vi "ReadTriggered.vi"(8 "error in (no error)":errorcluster, 10 "Keep last record only":bool, 11 "Scope5785_six_channel":refnum<class "Scope5782_six_channel.lvclass">) -> (0 "error out":errorcluster, 1 "#elements":i32, 2 "Data":dbl[][](array[numeric]), 3 "Scope5785_six_channel Out":refnum<class "Scope5782_six_channel.lvclass">)   [LabVIEW 2018, in "Scope5782_six_channel.lvclass"]
uses:
  Scope5782_six_channel.lvclass
  FpgaRef/FpgaRef5761/FpgaRef5761.lvclass
  FpgaRef/FpgaRef5782/FpgaRef5782.lvclass
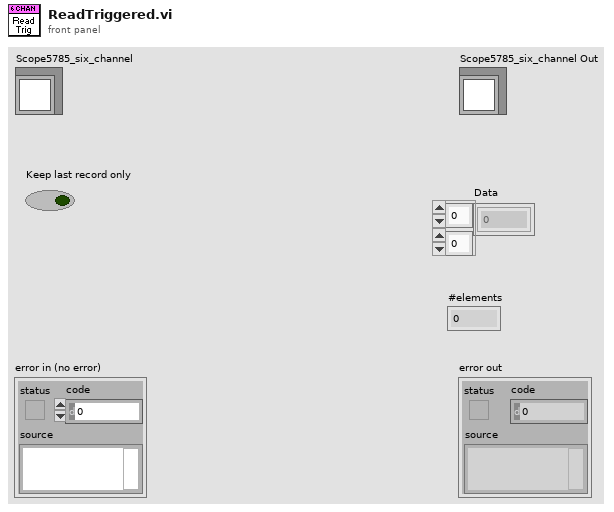
[diagram p1: front panel]
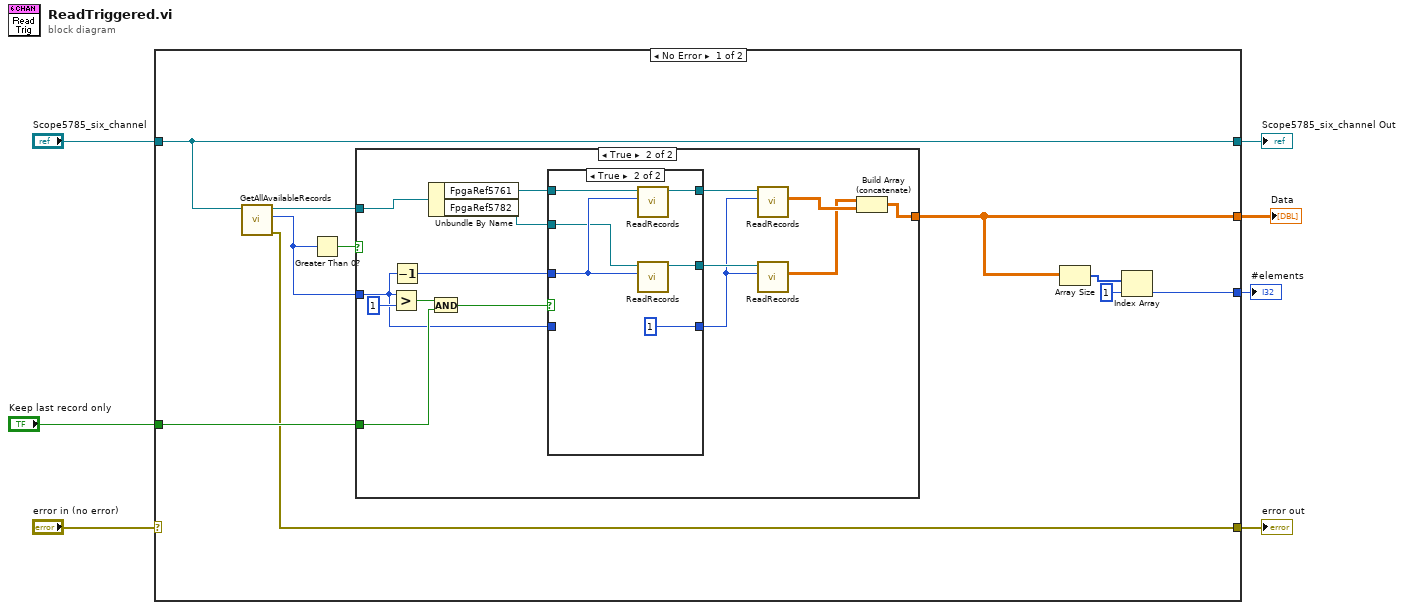
[diagram p0: block diagram]
diagram:
  n1 = case shown="No Error" "error in (no error)" {
    selector: "error in (no error)" -> [_ w43]
    tunnel: [w8 w43] -> w6
    tunnel: [w17 w42] -> w4
    tunnel: "Scope5785_six_channel" -> [w17 w42]
    tunnel: "Keep last record only" -> [w14 _]
    tunnel: [w12 _] -> w2
    tunnel: [w9 _] -> w1
    frame No Error {
      n2 = call-dynamic "GetAllAvailableRecords.vi"("Scope5785_six_channel"=w17) -> ("error out"=w8:errorcluster, "Available records"=w13:i32, "Scope5761 out"=w15:refnum<class "Scope5782_six_channel.lvclass">)  [unwired: 8 in]
      n3 = Greater Than 0?(x=w13) -> (x > 0?=w16:bool)
      n4 = case shown="True" w16 {
        tunnel: w15 -> [_ w27]
        tunnel: w14 -> [_ w30]
        tunnel: w13 -> [_ w24]
        tunnel: [_ w19] -> w12
        frame False {
        }
        frame True {
          n5 = Greater?(x=w24, y=1) -> (0:w31:bool)
          n6 = Decrement(x=w24) -> (x-1=w28:i32)
          n7 = Unbundle By Name(w27) -> ("FpgaRef5761"=w26:refnum<class "FpgaRef5761.lvclass">, "FpgaRef5782"=w25:refnum<class "FpgaRef5782.lvclass">)
          n8 = And(x=w31, y=w30) -> (x .and. y?=w29:bool)
          n9 = case shown="True" w29 {
            tunnel: w28 -> [_ w41]
            tunnel: w26 -> [w34 w40]
            tunnel: w25 -> [w33 w39]
            tunnel: [w34 w38] -> w23
            tunnel: [w33 w37] -> w22
            tunnel: [w35 1 ("y")] -> w21
            tunnel: w24 -> [w35 _]
            frame False {
            }
            frame True {
              n10 = call-dynamic "ReadRecords.vi"("Num records to read"=w41, "FpgaRef5761 In"=w40) -> ("FpgaRef5761 Out"=w38:refnum<class "FpgaRef5761.lvclass">)  [unwired: 7 in, 2 out]
              n11 = call-dynamic "ReadRecords.vi"("Num records to read"=w41, "FpgaRef5782 in"=w39) -> ("FpgaRef5782 out"=w37:refnum<class "FpgaRef5782.lvclass">)  [unwired: 7 in, 2 out]
            }
          }
          n12 = call-dynamic "ReadRecords.vi"("Num records to read"=w21, "FpgaRef5761 In"=w23) -> ("Data"=w20:dbl[][])  [unwired: 7 in, 2 out]
          n13 = call-dynamic "ReadRecords.vi"("Num records to read"=w21, "FpgaRef5782 in"=w22) -> ("Data"=w18:dbl[][])  [unwired: 7 in, 2 out]
          n14 = Build Array (concatenate)(w18, w20) -> (w19:dbl[][])
        }
      }
      n15 = Array Size(array=w12) -> (size(s)=w11:i32[])
      n16 = Index Array(array=w11, index=1) -> (element=w9:i32)
    }
    frame Error {
    }
  }
  "error out" <- w6
  "Scope5785_six_channel Out" <- w4
  "Data" <- w2
  "#elements" <- w1
